vi "CalculatePMAQI.vi"(8 "error in (no error)":errorcluster, 11 "Counts per Bin":dbl[](array[numeric])) -> (0 "error out":errorcluster, 3 "AQIPM cluster":T1)   [LabVIEW 2013]
doc: "Use this template to build a VI to use as a subVI."
uses:
  GRIMMAQIPM.ctl
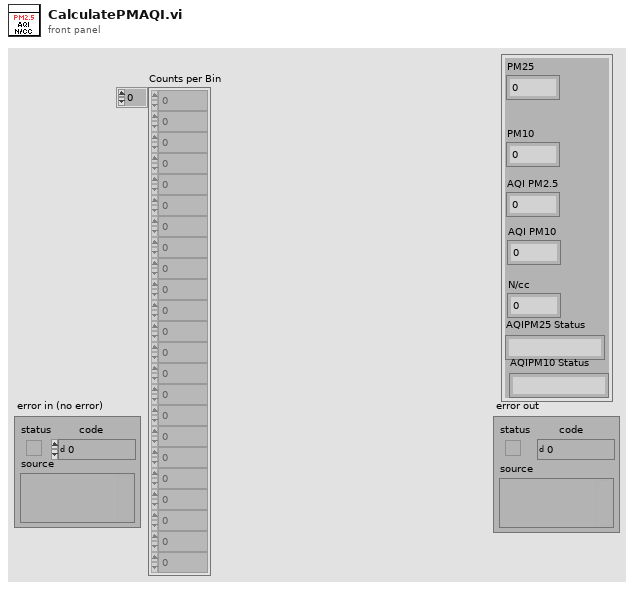
[diagram p1: front panel]
types:
  T1 = typedef "GRIMMAQIPM.ctl" = cluster{"PM25":dbl, "PM10":dbl, "AQI PM2.5":dbl, "N/cc":dbl, "AQI PM10":dbl, "AQIPM25 Status":string, "AQIPM10 Status":string}
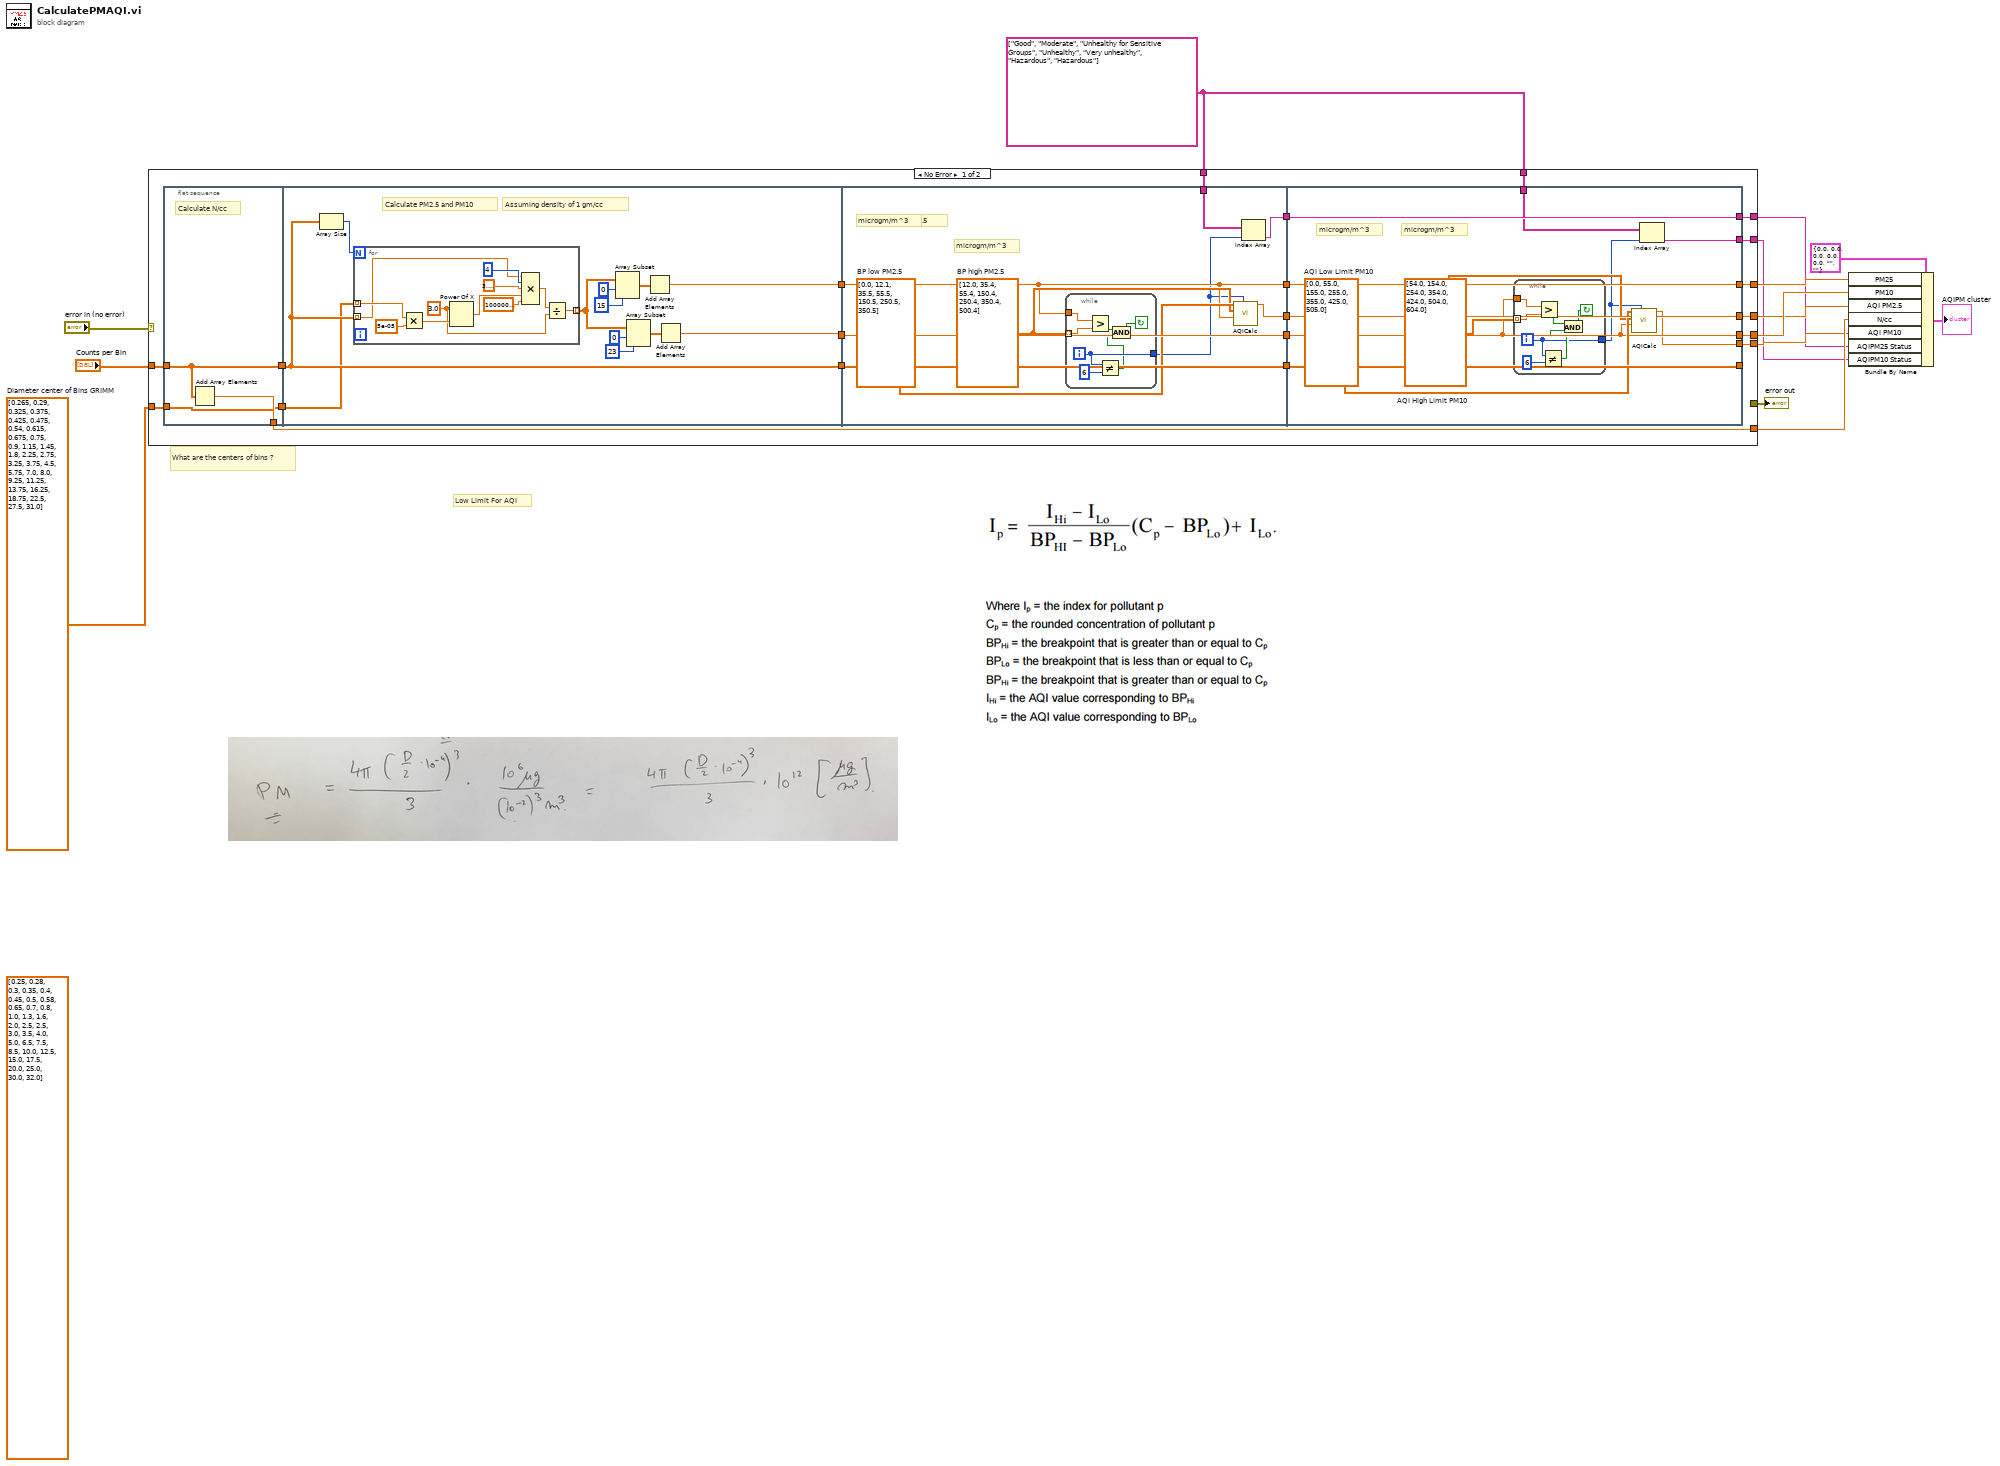
[diagram p0: block diagram]
diagram:
  w10 = string[] ["Good", "Moderate", "Unhealthy for Sensitive Groups", "Unhealthy", "Very unhealthy", "Hazardous", "Hazardous"]
  w11 = dbl[] [0.265, 0.29, 0.325, 0.375, 0.425, 0.475, 0.54, 0.615, 0.675, 0.75, 0.9, 1.15, 1.45, 1.8, 2.25, 2.75, 3.25, 3.75, 4.5, 5.75, 7.0, 8.0, 9.25, 11.25, 13.75, 16.25, 18.75, 22.5, 27.5, 31.0]  # Diameter center of Bins GRIMM
  (unwired) dbl[] [0.25, 0.28, 0.3, 0.35, 0.4, 0.45, 0.5, 0.58, 0.65, 0.7, 0.8, 1.0, 1.3, 1.6, 2.0, 2.5, 2.5, 3.0, 3.5, 4.0, 5.0, 6.5, 7.5, 8.5, 10.0, 12.5, 15.0, 17.5, 20.0, 25.0, 30.0, 32.0] ("Threshold Bin size")
  # "Low Limit For AQI"
  # "What are the centers of bins ?"
  n1 = case shown="No Error" "error in (no error)" {
    selector: "error in (no error)" -> [_ w96]
    tunnel: [_ w96] -> w13
    tunnel: "Counts per Bin" -> [w35 _]
    tunnel: [w34 _] -> w5
    tunnel: w11 -> [w31 _]
    tunnel: [w30 _] -> w8
    tunnel: [w29 _] -> w7
    tunnel: [w25 _] -> w6
    tunnel: [w20 _] -> w4
    tunnel: w10 -> [w19 _]
    tunnel: [w17 _] -> w3
    tunnel: w10 -> [w16 _]
    tunnel: [w15 _] -> w2
    frame No Error {
      n2 = flat-sequence {
        tunnel: w35 -> [w37]
        tunnel: [w38] -> w34
        tunnel: [w37] -> w33
        tunnel: [w36] -> w32
        tunnel: w31 -> [w36]
        tunnel: w33 -> [w49]
        tunnel: w32 -> [w39]
        tunnel: [w49] -> w28
        tunnel: [w45] -> w27
        tunnel: [w40] -> w26
        tunnel: w28 -> [w70]
        tunnel: w27 -> [w66]
        tunnel: w26 -> [w69]
        tunnel: [w70] -> w24
        tunnel: [w66] -> w23
        tunnel: [w69] -> w22
        tunnel: [w65] -> w21
        tunnel: w19 -> [w64]
        tunnel: [w62] -> w18
        tunnel: [w86] -> w25
        tunnel: [w83] -> w29
        tunnel: [w87] -> w30
        tunnel: [w88] -> _
        tunnel: w24 -> [w88]
        tunnel: w23 -> [w87]
        tunnel: w22 -> [w83]
        tunnel: w21 -> [w86]
        tunnel: [w82] -> w20
        tunnel: w18 -> [w81]
        tunnel: [w81] -> w17
        tunnel: w16 -> [w80]
        tunnel: [w78] -> w15
        frame #0 {
          # "Calculate N/cc"
          n3 = Add Array Elements(numeric array=w37) -> (sum=w38:dbl)
        }
        frame #1 {
          # "Assuming density of 1 gm/cc"
          # "Calculate PM2.5 and PM10"
          n4 = Array Size(array=w49) -> (size(s)=w50:i32)
          n5 = for {
            N: w50 -> [_]
            tunnel: w49 -> [w51] mode=indexing
            tunnel: [w54] -> w41 mode=indexing
            tunnel: w39 -> [w52] mode=indexing
            w53 = 3.0
            n6 = Multiply(x=w52, y=5e-05) -> (x*y=w58:dbl)
            n7 = Power Of X(1:w58, 2:w53) -> (0:w57:dbl)
            n8 = Compound Arithmetic op=MULTIPLY(w51, 4, 3.141592653589793, w57, 1000000000000.0) -> (w56:dbl)
            n9 = Divide(x=w56, y=w53) -> (x/y=w54:dbl)
          }
          n10 = Array Subset(array=w41, index=0, length=15) -> (w46:dbl[])
          n11 = Array Subset(array=w41, index=0, length=23) -> (w44:dbl[])
          n12 = Add Array Elements(numeric array=w46) -> (sum=w45:dbl)
          n13 = Add Array Elements(numeric array=w44) -> (sum=w40:dbl)
        }
        frame #2 {
          w67 = dbl[] [12.0, 35.4, 55.4, 150.4, 250.4, 350.4, 500.4]  # BP high PM2.5
          w68 = dbl[] [0.0, 12.1, 35.5, 55.5, 150.5, 250.5, 350.5]  # BP low PM2.5
          # "microgm/m^3"
          # "microgm/m^3"
          # "Calculate AQI PM2.5"
          n14 = while {
            tunnel: w67 -> [w76] mode=indexing
            tunnel: w66 -> [w77]
            tunnel: [w75] -> w63
            i -> [w75]
            stop <- w71 continue-if-true
            n15 = Greater?(x=w77, y=w76) -> (0:w73:bool)
            n16 = Not Equal?(x=w75, y=6) -> (x != y?=w72:bool)
            n17 = And(x=w73, y=w72) -> (x .and. y?=w71:bool)
          }
          n18 = call "AQICalc.vi"("ChosenRange"=w63, "PMMeasurement"=w66, "BP high PM"=w67, "BP low PM"=w68) -> ("AQI"=w65:dbl)  [unwired: 6 in, 1 out]
          n19 = Index Array(array=w64, index=w63) -> (element=w62:string)
        }
        frame #3 {
          w84 = dbl[] [54.0, 154.0, 254.0, 354.0, 424.0, 504.0, 604.0]  # AQI High Limit PM10
          w85 = dbl[] [0.0, 55.0, 155.0, 255.0, 355.0, 425.0, 505.0]  # AQI Low Limit PM10
          # "microgm/m^3"
          # "microgm/m^3"
          n20 = while {
            tunnel: w84 -> [w94] mode=indexing
            tunnel: w83 -> [w95]
            tunnel: [w89] -> w79
            i -> [w89]
            stop <- w90 continue-if-true
            n21 = Greater?(x=w95, y=w94) -> (0:w91:bool)
            n22 = Not Equal?(x=w89, y=6) -> (x != y?=w93:bool)
            n23 = And(x=w91, y=w93) -> (x .and. y?=w90:bool)
          }
          n24 = call "AQICalc.vi"("ChosenRange"=w79, "PMMeasurement"=w83, "BP high PM"=w84, "BP low PM"=w85) -> ("AQI"=w82:dbl)  [unwired: 6 in, 1 out]
          n25 = Index Array(array=w80, index=w79) -> (element=w78:string)
        }
      }
    }
    frame Error {
    }
  }
  "error out" <- w13
  n26 = Bundle By Name(cluster=T1 {"PM25"=0.0, "PM10"=0.0, "AQI PM2.5"=0.0, "N/cc"=0.0, "AQI PM10"=0.0, "AQIPM25 Status"="", "AQIPM10 Status"=""}, "PM25"=w8, "PM10"=w7, "AQI PM2.5"=w6, "N/cc"=w5, "AQI PM10"=w4, "AQIPM25 Status"=w3, "AQIPM10 Status"=w2) -> (→"AQIPM cluster":T1)
